vi "Oriantation Calculation.vi"(1 "Oriantation Info In":T1) -> (0 "Oriantation Info Out":T1)   [LabVIEW 2013]
uses:
  Oritentation Global.vi
  Camera/Camera Global.vi
panel:
  # "The Horizontal \nVector of the \nCamera Mounts\nDistance"
  # "The Horizontal \nVector of the \nCamera Mounts\nDistance"
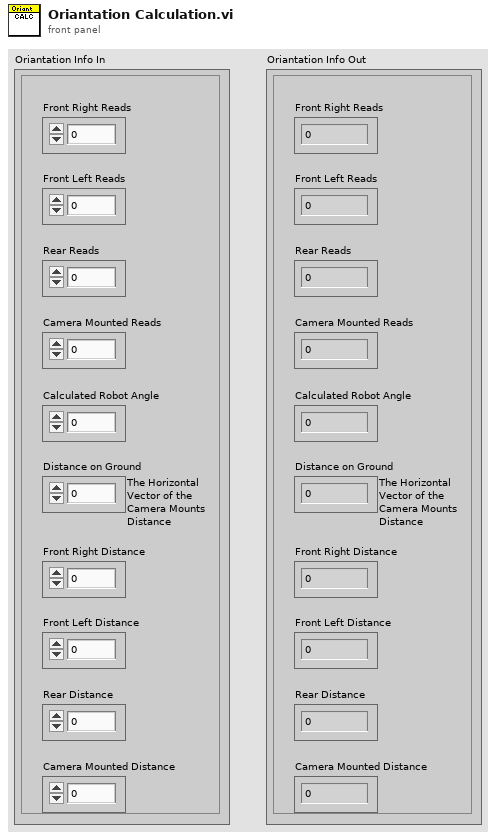
[diagram p1: front panel]
types:
  T1 = cluster{"Front Right Reads":dbl, "Front Left Reads ":dbl, "Rear Reads":dbl, "Camera Mounted Reads":dbl, "Calculated Robot Angle":dbl, "Distance on Ground":dbl, "Front Right Distance":dbl, "Front Left Distance":dbl, "Rear Distance":dbl, "Camera Mounted Distance":dbl}
  T2 = cluster{"Manual X Angle":dbl, "Manual Y Angle ":dbl, "Set X Angle":dbl, "Set Y Angle ":dbl, "Wanted X Angle":dbl, "Wanted Y Angle  ":dbl}
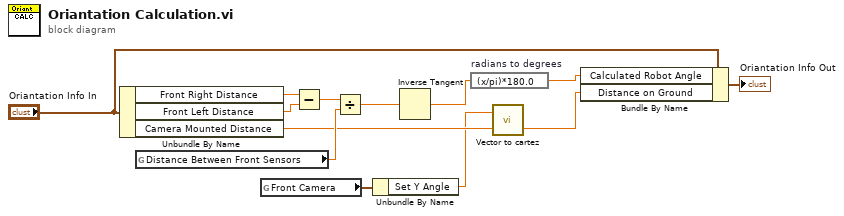
[diagram p0: block diagram]
diagram:
  n1 = Unbundle By Name("Oriantation Info In") -> ("Front Right Distance"=w11:dbl, "Front Left Distance"=w10:dbl, "Camera Mounted Distance"=w4:dbl)
  n2 = global read "Oritentation Global.vi" "Distance Between Front Sensors"() -> (w8:dbl)
  n3 = global read "Camera Global.vi" "Front Camera"() -> (w3:T2)
  n4 = Subtract(x=w11, y=w10) -> (x-y=w9:dbl)
  n5 = Divide(x=w9, y=w8) -> (x/y=w7:dbl)
  n6 = Unbundle By Name(w3) -> ("Set Y Angle"=w2:dbl)
  n7 = Inverse Tangent(1:w7) -> (0:w6:dbl)
  n8 = expression code="(x/pi)*180.0" "radians to degrees"(w6) -> (w5:dbl)
  n9 = call "Vector to cartez.vi"("Vector"=w4, "Angle [deg]"=w2) -> ("Length"=w1:dbl)  [unwired: 1 out]
  n10 = Bundle By Name(cluster="Oriantation Info In", "Calculated Robot Angle"=w5, "Distance on Ground"=w1) -> (→"Oriantation Info Out":T1)
